vi "Is Row Hidden.vi"(10 "Tag":string, 11 "TreeControl in":refnum<vi>) -> (3 "Hidden":bool)   [LabVIEW 2020, in "Output Sequencer.lvlib" / "Settings UI.lvclass"]
uses:
  Settings UI.lvclass
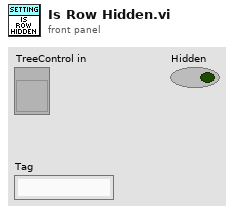
[diagram p1: front panel]
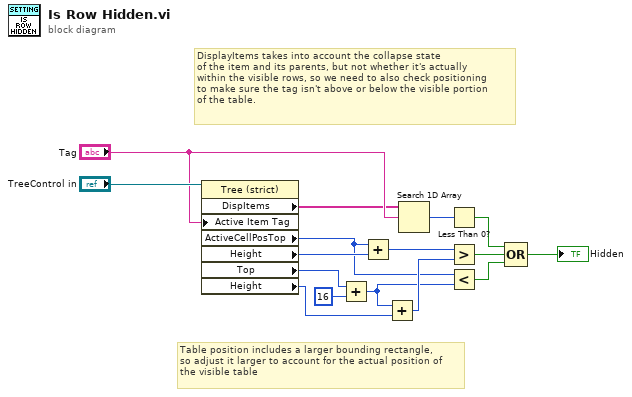
[diagram p0: block diagram]
diagram:
  # "DisplayItems takes into account the collapse state\nof the item and its parents, but not whether it's actually\nwithin the visible rows, so we need to also check positioning\nto make sure the tag isn't above or below the visible portion\nof the table."
  # "Table position includes a larger bounding rectangle,\nso adjust it larger to account for the actual position of\nthe visible table"
  n1 = property class="Tree (strict)"(reference="TreeControl in", "Active Item Tag"="Tag") -> ("DispItems"=w13:string[], "ActiveCellPosTop"=w3:i32, "Height"=w11:i32, "Top"=w8:i32, "Height"=w7:u32)  [unwired: 1 in, 2 out]
  n2 = Add(x=w8, y=16) -> (x+y=w2:i32)
  n3 = Add(x=w3, y=w11) -> (x+y=w10:i32)
  n4 = Add(x=w2, y=w7) -> (x+y=w6:u32)
  n5 = Search 1D Array(1D array=w13, element="Tag") -> (index of element=w12:i32)  [unwired: 1 in]
  n6 = Less Than 0?(x=w12) -> (x < 0?=w4:bool)
  n7 = Greater?(x=w10, y=w6) -> (0:w5:bool)
  n8 = Less?(x=w3, y=w2) -> (x < y?=w1:bool)
  n9 = Compound Arithmetic op=OR(w4, w5, w1) -> (→"Hidden":bool)
